vi "getError.vi"(8 "error":errorcluster, 11 "connection ID":refnum<k5>) -> (0 "error out":errorcluster, 2 "Output parameters":T1, 3 "connection ID out":refnum<k5>)   [LabVIEW 2016, in "amc_api.lvlib"]
doc: "Reads the statuses of the RT- and ethernet-connection.\n All return parameters follow the following logic:\n 0: no error occured since last reset\n 1: error is occurring at the moment\n 2: error occured in the past, but not at the moment\n 3: error is occurring at the moment and latched"
uses:
  amc_api.lvlib
panel:
  out "jsonRespIn":string
  out "JSON-response":string="{\"jsonrpc\":\"2.0\",\"method\":\"\",\"params\":[5,1.245,true,\"name\"],\"id\":\"1\"}"
  out "JSON request":string
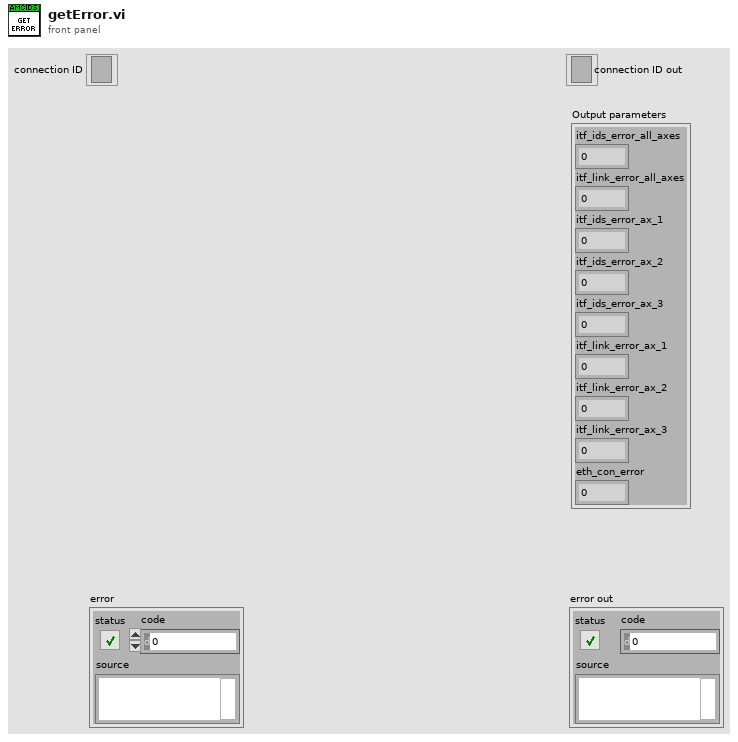
[diagram p1: front panel]
types:
  T1 = cluster{"itf_ids_error_all_axes":i32, "itf_link_error_all_axes":i32, "itf_ids_error_ax_1":i32, "itf_ids_error_ax_2":i32, "itf_ids_error_ax_3":i32, "itf_link_error_ax_1":i32, "itf_link_error_ax_2":i32, "itf_link_error_ax_3":i32, "eth_con_error":i32}
  T2 = cluster{"jsonrpc":string, "method":string, "params":string[], "id":string, "api":i32, "pid":string}
  T3 = enum16{"Standard", "Buffered", "CRLF", "Immediate"}
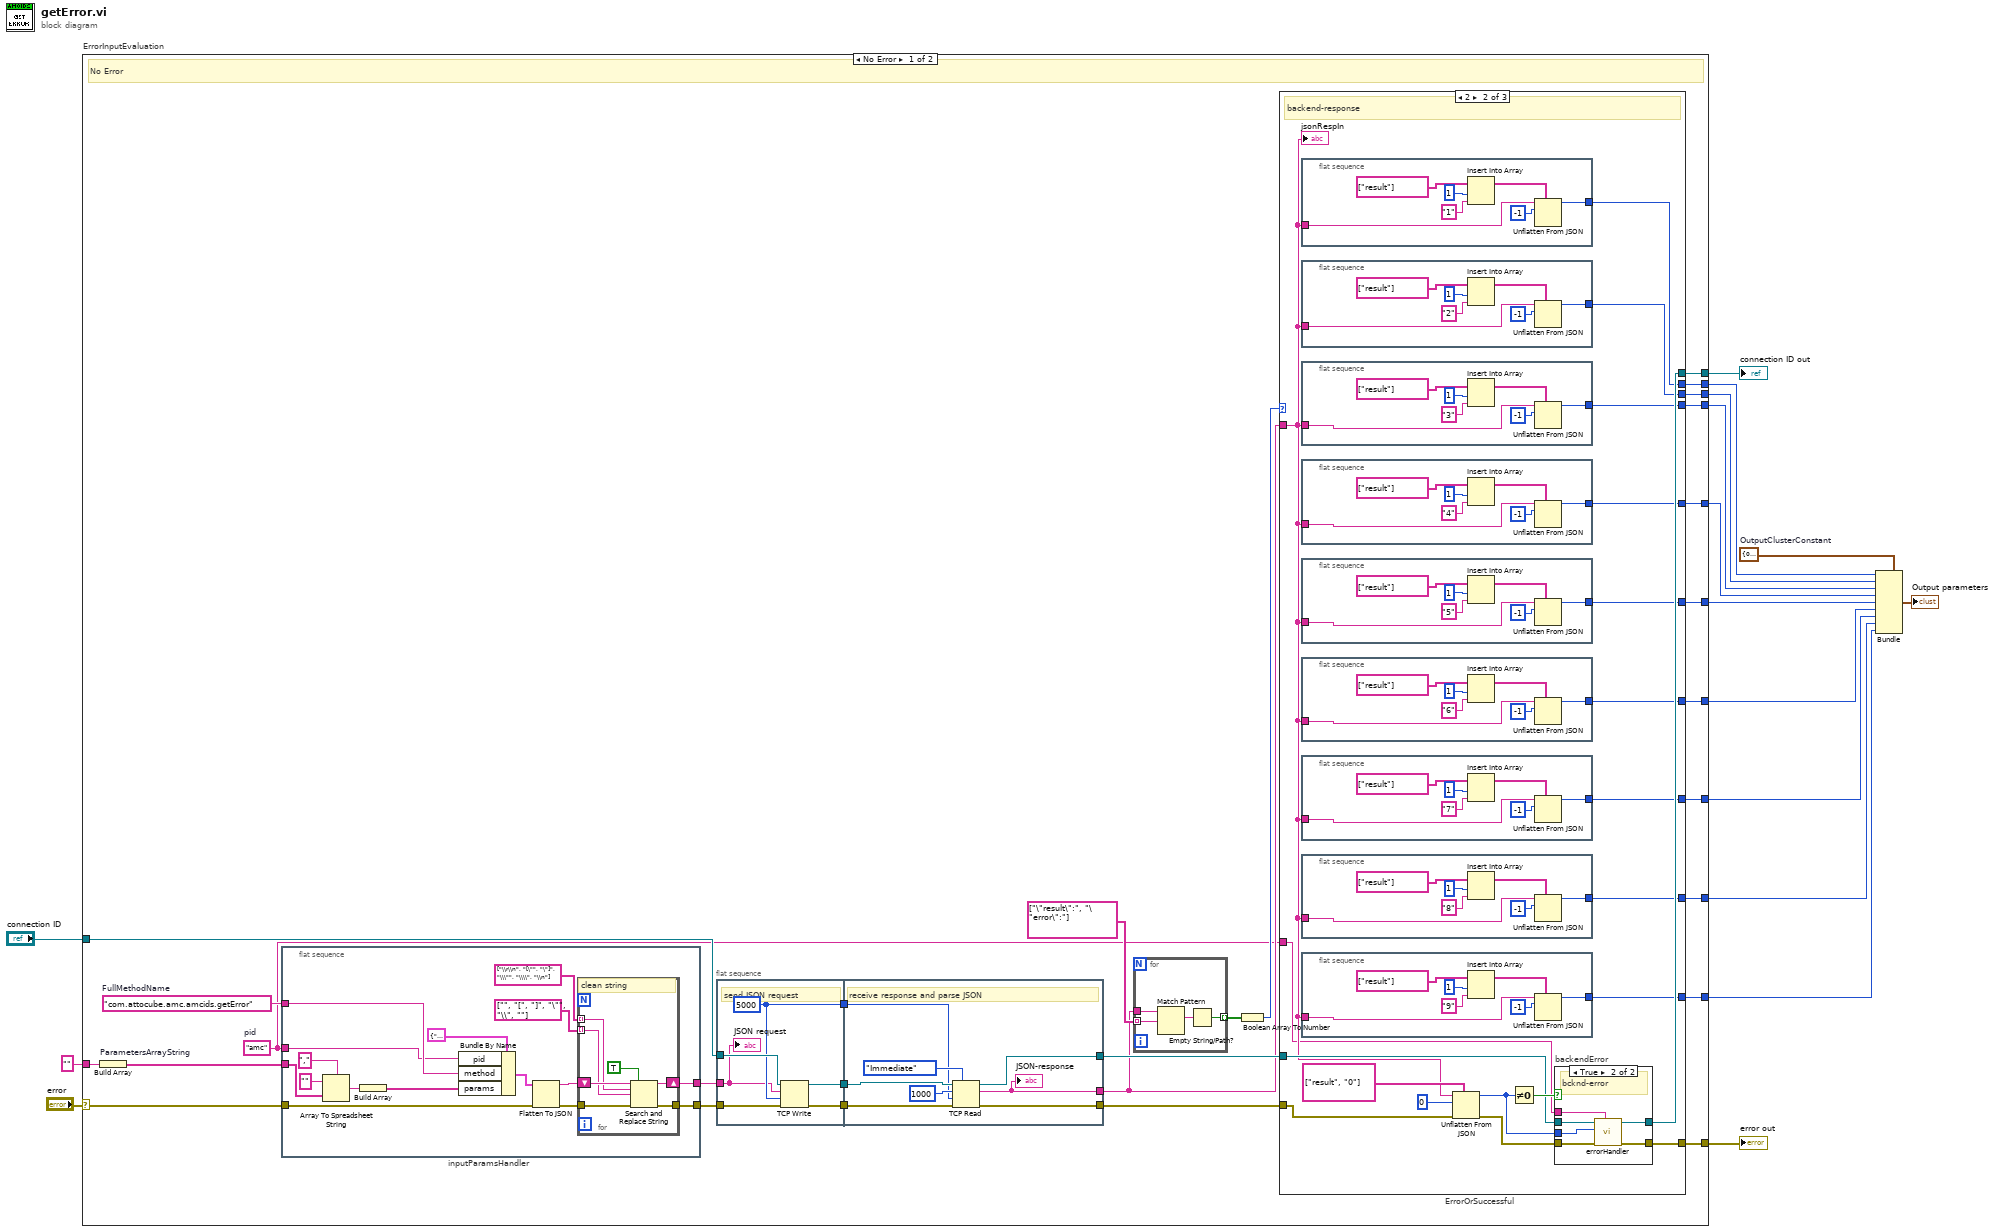
[diagram p0: block diagram]
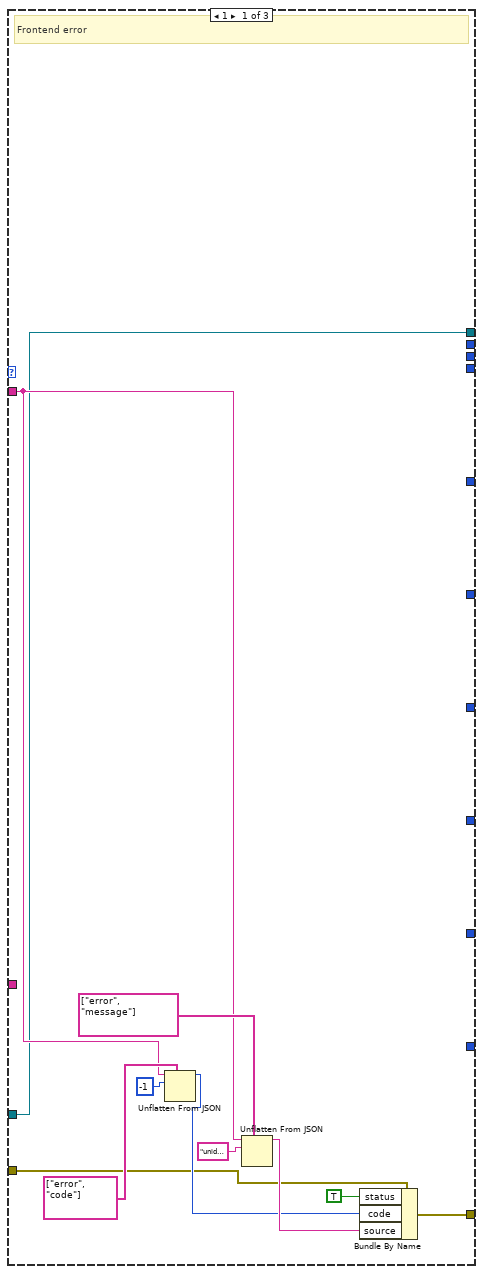
[diagram p2: hidden frame]
diagram:
  w15 = T1 {"itf_ids_error_all_axes"=0, "itf_link_error_all_axes"=0, "itf_ids_error_ax_1"=0, "itf_ids_error_ax_2"=0, "itf_ids_error_ax_3"=0, "itf_link_error_ax_1"=0, "itf_link_error_ax_2"=0, "itf_link_error_ax_3"=0, "eth_con_error"=0}  # OutputClusterConstant
  n1 = case "ErrorInputEvaluation" shown="No Error" "error" {
    selector: "error" -> [w31 w190]
    tunnel: "connection ID" -> [w41 w191]
    tunnel: [w33 w190] -> w14
    tunnel: [w34 w191] -> w13
    tunnel: "" -> [w26 _]
    tunnel: [w25 _] -> w10
    tunnel: [w24 _] -> w9
    tunnel: [w23 _] -> w8
    tunnel: [w22 _] -> w7
    tunnel: [w21 _] -> w6
    tunnel: [w20 _] -> w5
    tunnel: [w19 _] -> w4
    tunnel: [w18 _] -> w3
    tunnel: [w17 _] -> w2
    frame No Error {
      w27 = "amc"  # pid
      w32 = "com.attocube.amc.amcids.getError"  # FullMethodName
      # "No Error"
      n2 = Build Array "ParametersArrayString"(w26) -> (w30:string[])
      n3 = flat-sequence "inputParamsHandler" {
        tunnel: [w50] -> w29
        tunnel: w30 -> [w56]
        tunnel: w31 -> [w55]
        tunnel: [w52] -> w28
        tunnel: w32 -> [w46]
        tunnel: w27 -> [w45]
        frame #0 {
          n4 = Array To Spreadsheet String(delimiter (Tab)=",", array=w56, 3:"" ("format string")) -> (spreadsheet string=w58:string)
          n5 = Build Array "Build Array"(w58) -> (w47:string[])
          n6 = Bundle By Name(cluster=T2 {"jsonrpc"="2.0", "method"="com.attocube.amc.res.setRESReadOutFreq", "params"=[], "id"="1", "api"=2, "pid"=""}, "pid"=w45, "method"=w46, "params"=w47) -> (w57:T2)
          n7 = Flatten To JSON(anything=w57, error in (no error)=w55) -> (JSON string=w51:string, 11:w53:errorcluster)  [unwired: 1 in]
          n8 = for {
            tunnel: string[] ["\\r\\n", "[\"", "\"]", "\\\"", "\\\\", "\\n"] ("search string") -> [w64] mode=indexing
            tunnel: string[] ["", "[", "]", "\"", "\\", ""] ("replace string (\"\")") -> [w63] mode=indexing
            shift-right: [w66] -> w50
            shift-left: w51 -> [w65]
            tunnel: w53 -> [w62]
            tunnel: [w61] -> w52
            # "clean string"
            n9 = Search and Replace String(replace all?=TRUE ("replace all? (F)"), input string=w65, search string=w64, replace string=w63, error in=w62) -> (result string=w66:string, error out=w61:errorcluster)  [unwired: 3 in, 2 out]
          }
        }
      }
      n10 = flat-sequence {
        tunnel: w41 -> [w181]
        tunnel: [w179] -> w44
        tunnel: [w180] -> w43
        tunnel: w28 -> [w176]
        tunnel: [w178] -> w42
        tunnel: w29 -> [w177]
        tunnel: [w185] -> w37
        tunnel: w44 -> [w187]
        tunnel: w43 -> [w186]
        tunnel: [w183] -> w36
        tunnel: w42 -> [w184]
        tunnel: [w182] -> w35
        frame #0 {
          w178 = 5000 ("timeout ms (25000)")
          # "send JSON request"
          n11 = TCP Write(connection ID=w181, data in=w177, error in (no error)=w176, 9:w178) -> (connection ID out=w179:refnum<k5>, error out=w180:errorcluster)  [unwired: 1 out]
          "JSON request" <- w177
        }
        frame #1 {
          # "receive response and parse JSON"
          n12 = TCP Read(connection ID=w187, bytes to read=1000, error in (no error)=w186, 7:T3."Immediate" ("mode (standard)"), 9:w184) -> (connection ID out=w185:refnum<k5>, data out=w182:string, error out=w183:errorcluster)
          "JSON-response" <- w182
        }
      }
      n13 = for {
        tunnel: string[] ["\"result\":", "\"error\":"] ("path") -> [w70] mode=indexing
        tunnel: [w68] -> w39 mode=indexing
        tunnel: w35 -> [w71]
        n14 = Match Pattern(string=w71, regular expression=w70) -> (match substring=w69:string)  [unwired: 1 in, 3 out]
        n15 = Empty String/Path?(string/path=w69) -> (empty?=w68:bool)
      }
      n16 = Boolean Array To Number(Boolean array=w39) -> (number=w38:u32)
      n17 = case "ErrorOrSuccessful" shown="2" w38 {
        tunnel: w35 -> [w74 w93 _]
        tunnel: w37 -> [w72 w96 w175]
        tunnel: [w72 w95 w175] -> w34
        tunnel: [w75 w94 w174] -> w33
        tunnel: w36 -> [w73 w97 w174]
        tunnel: w27 -> [_ w92 _]
        tunnel: [_ w91 _] -> w25
        tunnel: [_ w90 _] -> w24
        tunnel: [_ w89 _] -> w23
        tunnel: [_ w88 _] -> w22
        tunnel: [_ w87 _] -> w21
        tunnel: [_ w86 _] -> w20
        tunnel: [_ w85 _] -> w19
        tunnel: [_ w84 _] -> w18
        tunnel: [_ w83 _] -> w17
        frame 1 {
          # "Frontend error"
          n18 = Unflatten From JSON(path=string[] ["error", "code"], JSON string=w74, type and defaults=-1) -> (value=w81:i32)  [unwired: 4 in, 1 out]
          n19 = Unflatten From JSON(path=string[] ["error", "message"], JSON string=w74, type and defaults="unidentified error") -> (value=w82:string)  [unwired: 4 in, 1 out]
          n20 = Bundle By Name(cluster=w73, "status"=TRUE, "code"=w81, "source"=w82) -> (w75:errorcluster)
        }
        frame 2 {
          # "backend-response"
          n21 = flat-sequence "out_integer" {
            tunnel: w93 -> [w161]
            tunnel: [w159] -> w91
            frame #0 {
              n22 = Insert Into Array(array=string[] ["result"] ("path"), index=1, new element="1" ("idx")) -> (w163:string[])
              n23 = Unflatten From JSON(path=w163, JSON string=w161, type and defaults=-1 ("index")) -> (value=w159:i32)  [unwired: 4 in, 1 out]
            }
          }
          n24 = flat-sequence "out_integer" {
            tunnel: w93 -> [w154]
            tunnel: [w152] -> w90
            frame #0 {
              n25 = Insert Into Array(array=string[] ["result"] ("path"), index=1, new element="2" ("idx")) -> (w156:string[])
              n26 = Unflatten From JSON(path=w156, JSON string=w154, type and defaults=-1 ("index")) -> (value=w152:i32)  [unwired: 4 in, 1 out]
            }
          }
          n27 = flat-sequence "out_integer" {
            tunnel: w93 -> [w147]
            tunnel: [w145] -> w89
            frame #0 {
              n28 = Insert Into Array(array=string[] ["result"] ("path"), index=1, new element="3" ("idx")) -> (w149:string[])
              n29 = Unflatten From JSON(path=w149, JSON string=w147, type and defaults=-1 ("index")) -> (value=w145:i32)  [unwired: 4 in, 1 out]
            }
          }
          n30 = flat-sequence "out_integer" {
            tunnel: w93 -> [w140]
            tunnel: [w138] -> w88
            frame #0 {
              n31 = Insert Into Array(array=string[] ["result"] ("path"), index=1, new element="4" ("idx")) -> (w142:string[])
              n32 = Unflatten From JSON(path=w142, JSON string=w140, type and defaults=-1 ("index")) -> (value=w138:i32)  [unwired: 4 in, 1 out]
            }
          }
          n33 = flat-sequence "out_integer" {
            tunnel: w93 -> [w133]
            tunnel: [w131] -> w87
            frame #0 {
              n34 = Insert Into Array(array=string[] ["result"] ("path"), index=1, new element="5" ("idx")) -> (w135:string[])
              n35 = Unflatten From JSON(path=w135, JSON string=w133, type and defaults=-1 ("index")) -> (value=w131:i32)  [unwired: 4 in, 1 out]
            }
          }
          n36 = flat-sequence "out_integer" {
            tunnel: w93 -> [w126]
            tunnel: [w124] -> w86
            frame #0 {
              n37 = Insert Into Array(array=string[] ["result"] ("path"), index=1, new element="6" ("idx")) -> (w128:string[])
              n38 = Unflatten From JSON(path=w128, JSON string=w126, type and defaults=-1 ("index")) -> (value=w124:i32)  [unwired: 4 in, 1 out]
            }
          }
          n39 = flat-sequence "out_integer" {
            tunnel: w93 -> [w119]
            tunnel: [w117] -> w85
            frame #0 {
              n40 = Insert Into Array(array=string[] ["result"] ("path"), index=1, new element="7" ("idx")) -> (w121:string[])
              n41 = Unflatten From JSON(path=w121, JSON string=w119, type and defaults=-1 ("index")) -> (value=w117:i32)  [unwired: 4 in, 1 out]
            }
          }
          n42 = flat-sequence "out_integer" {
            tunnel: w93 -> [w112]
            tunnel: [w110] -> w84
            frame #0 {
              n43 = Insert Into Array(array=string[] ["result"] ("path"), index=1, new element="8" ("idx")) -> (w114:string[])
              n44 = Unflatten From JSON(path=w114, JSON string=w112, type and defaults=-1 ("index")) -> (value=w110:i32)  [unwired: 4 in, 1 out]
            }
          }
          n45 = flat-sequence "out_integer" {
            tunnel: w93 -> [w105]
            tunnel: [w103] -> w83
            frame #0 {
              n46 = Insert Into Array(array=string[] ["result"] ("path"), index=1, new element="9" ("idx")) -> (w107:string[])
              n47 = Unflatten From JSON(path=w107, JSON string=w105, type and defaults=-1 ("index")) -> (value=w103:i32)  [unwired: 4 in, 1 out]
            }
          }
          n48 = Unflatten From JSON(path=string[] ["result", "0"], JSON string=w93, type and defaults=0, error in (no error)=w97) -> (value=w102:i32, error out=w100:errorcluster)  [unwired: 3 in]
          n49 = Not Equal To 0?(x=w102) -> (x != 0?=w101:bool)
          n50 = case "backendError" shown="True" w101 {
            tunnel: w102 -> [_ w173]
            tunnel: w100 -> [w167 w172]
            tunnel: [w166 w171] -> w95
            tunnel: [w167 w170] -> w94
            tunnel: w96 -> [w166 w169]
            tunnel: w92 -> [_ w168]
            frame False {
              # "successful"
            }
            frame True {
              # "bcknd-error"
              n51 = call "errorHandler.vi"("pid"=w168, "error in"=w172, "errNbr"=w173, "connection ID"=w169) -> ("error out 2"=w170:errorcluster, "connection ID out"=w171:refnum<k5>)  [unwired: 6 in]
            }
          }
          "jsonRespIn" <- w93
        }
        frame Default {
          # "NoResponse"
        }
      }
    }
    frame Error {
      # "Error"
    }
  }
  "error out" <- w14
  "connection ID out" <- w13
  n52 = Bundle ("BundleOutputs")(cluster=w15, "itf_ids_error_all_axes"=w10, "itf_link_error_all_axes"=w9, "itf_ids_error_ax_1"=w8, "itf_ids_error_ax_2"=w7, "itf_ids_error_ax_3"=w6, "itf_link_error_ax_1"=w5, "itf_link_error_ax_2"=w4, "itf_link_error_ax_3"=w3, "eth_con_error"=w2) -> (→"Output parameters":T1)
